vi "cb_mouseDblCk.vi"(4 "user param":refnum<vi>[](array[refnum]), 5 "이벤트 데이터":cluster{"sender":refnum<k24>, "e":refnum<k24>}, 6 "컨트롤 참조":refnum<k24>, 7 "이벤트 일반 데이터":cluster{"이벤트 소스":i32, "이벤트 타입":u32, "타임스탬프":u32}) -> ()   [LabVIEW 2019]
uses:
  dll/GMap.NET.WindowsForms.dll
  System.Windows.Forms
  gmap_fgv-cmd.ctl
  marker_info.ctl
  dll/GMap.NET.Core.dll
  System.Drawing
panel:
  out "type":i32(ring)=32 items=["none", "arrow", "blue", "blue_small", "blue_dot", "blue_pushpin", "brown_small", "gray_small", "green", "green_small", "green_dot", "green_pushpin", "green_big_go", "yellow", "yellow_small", "yellow_dot", "yellow_big_pause", "yellow_pushpin", "lightblue", "lightblue_dot", "lightblue_pushpin", "orange", "orange_small", "orange_dot", "pink", "pink_dot", "pink_pushpin", "purple", "purple_small", "purple_dot", "purple_pushpin", "red", "red_small", "red_dot", "red_pushpin", "red_big_stop", "black_small", "white_small"]
  out "Contains":bool
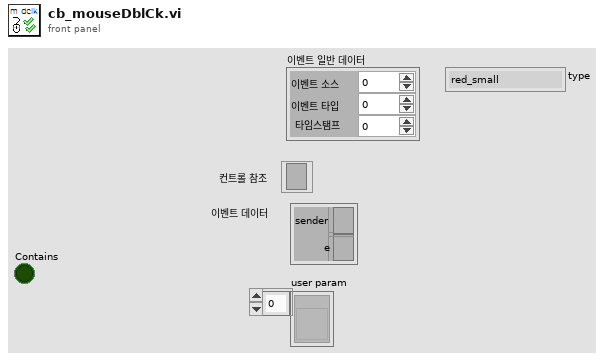
[diagram p1: front panel]
types:
  T1 = typedef "marker_info.ctl" = cluster{"arrLatLngActv":dbl[], "type":i32}
  T2 = typedef "gmap_fgv-cmd.ctl" = enum16{"marker type change", "save_image", "coll of points", "zoom n center markers", "add overlay reference", "read", "zoom", "set position by keyword", "set map provider", "map provider update", "create", "add marker", "clear marker", "close"}
  T3 = cluster{"MouseLat":refnum<vi>, "MouseLog":refnum<vi>, "MouseLat_DbClk":refnum<vi>, "MouseLog_DbClk":refnum<vi>, "PinDropLat_DblClk":refnum<vi>, "zoom":refnum<vi>}
  T4 = enum16{"none", "arrow", "blue", "blue_small", "blue_dot", "blue_pushpin", "brown_small", "gray_small", "green", "green_small", "green_dot", "green_pushpin", "green_big_go", "yellow", "yellow_small", "yellow_dot", "yellow_big_pause", "yellow_pushpin", "lightblue", "lightblue_dot", "lightblue_pushpin", "orange", "orange_small", "orange_dot", "pink", "pink_dot", "pink_pushpin", "purple", "purple_small", "purple_dot", "purple_pushpin", "red", "red_small", "red_dot", "red_pushpin", "red_big_stop", "black_small", "white_small"}
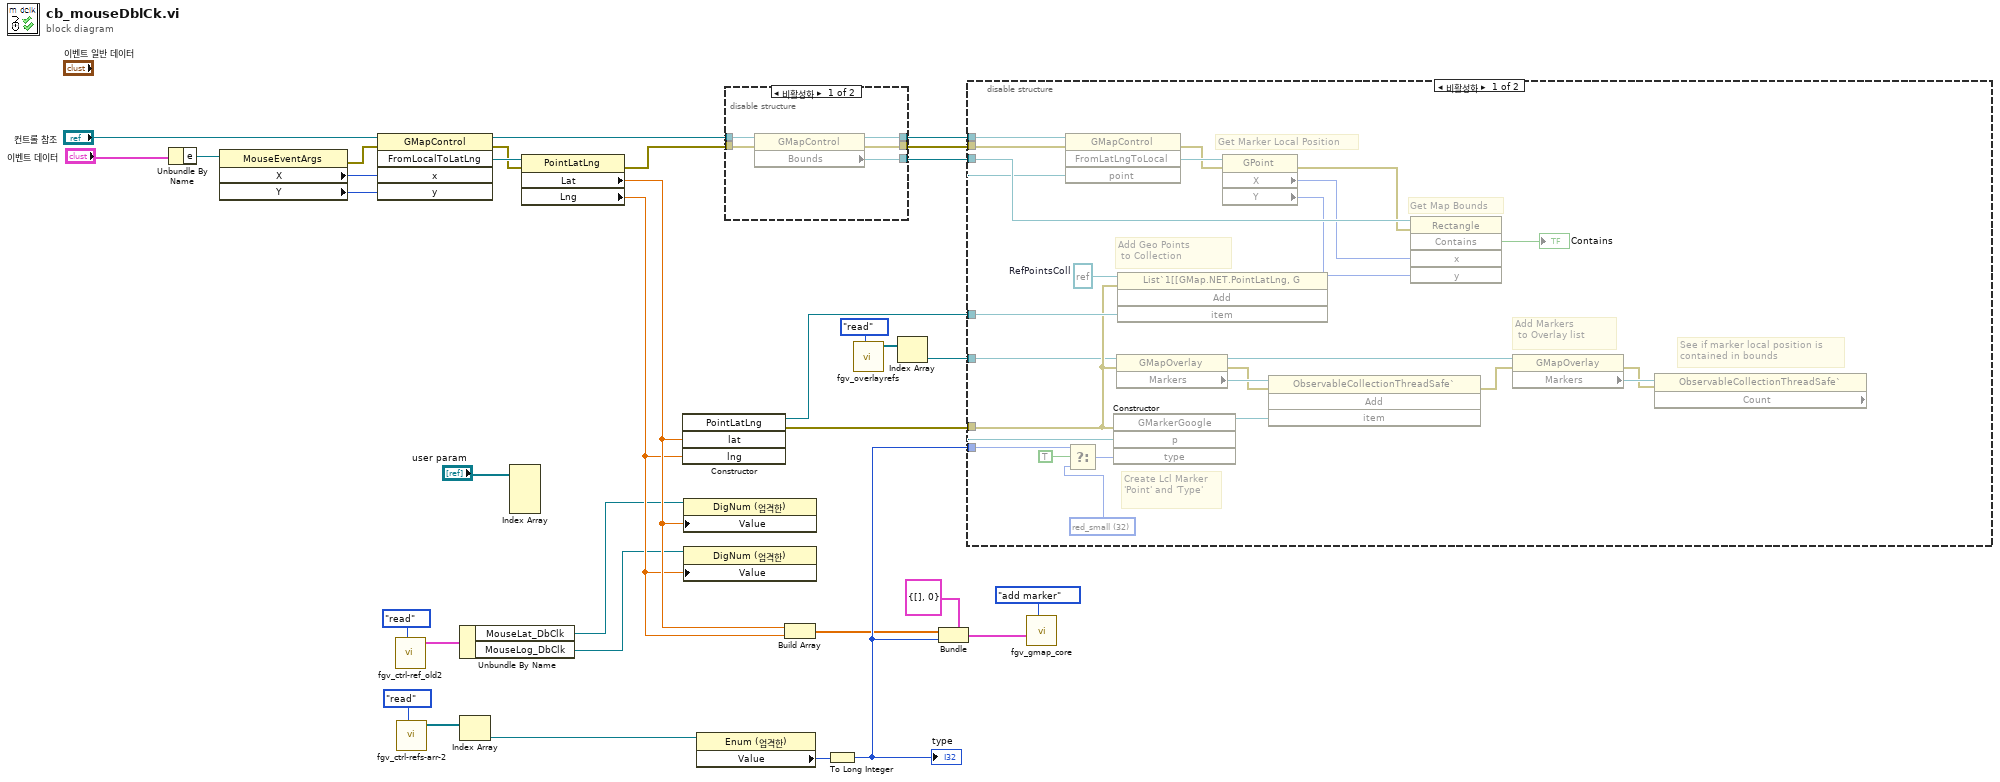
[diagram p0: block diagram]
diagram:
  n1 = Unbundle By Name("이벤트 데이터") -> ("e"=w24:refnum<k24>)
  n2 = property class="MouseEventArgs"(reference=w24) -> (error out=w20:errorcluster, "X"=w26:i32, "Y"=w25:i32)  [unwired: 1 in, 1 out]
  n3 = invoke class="GMapControl" method="FromLocalToLatLng"(reference="컨트롤 참조", error in=w20, "x"=w26, "y"=w25) -> (reference out=w17:refnum<k24>, error out=w19:errorcluster, "FromLocalToLatLng"=w23:refnum<k24>)  [unwired: 1 in, 2 out]
  n4 = call "fgv_ctrl-ref_old2.vi"("cmd"=enum16{"read", "write"}."read") -> ("ref out"=w1:T3)  [unwired: 10 in]
  n5 = call "fgv_ctrl-refs-arr-2.vi"("cmd"=enum16{"read", "write"}."read") -> ("ref out"=w4:refnum<vi>[])  [unwired: 10 in]
  n6 = Unbundle By Name(w1) -> ("MouseLat_DbClk"=w7:refnum<vi>, "MouseLog_DbClk"=w6:refnum<vi>)
  n7 = Index Array(array=w4) -> (element=w3:refnum<vi>)  [unwired: 1 in]
  n8 = Index Array(array="user param") -> ()  [unwired: 4 in, 4 out]
  n9 = property class="PointLatLng"(reference=w23, error in=w19) -> (error out=w18:errorcluster, "Lat"=w11:dbl, "Lng"=w10:dbl)  [unwired: 1 out]
  n10 = constructor class="PointLatLng"("lat"=w11, "lng"=w10) -> (reference out=w30:refnum<k24>, error out=w29:errorcluster)  [unwired: 3 in, 3 out]
  n11 = property class="DigNum (엄격한)"(reference=w7, "Value"=w11) -> ()  [unwired: 1 in, 2 out]
  n12 = property class="DigNum (엄격한)"(reference=w6, "Value"=w10) -> ()  [unwired: 1 in, 2 out]
  n13 = property class="Enum (엄격한)"(reference=w3) -> ("Value"=w15:T4)  [unwired: 1 in, 2 out]
  n14 = disable-structure shown="비활성화" {
    disable-tunnel: [w39 _] -> w33
    disable-tunnel: [w38 _] -> w32
    disable-tunnel: [w37 _] -> w31
    disable-tunnel: w18 -> [w36 _]
    disable-tunnel: w17 -> [w35 _]
    frame Disabled {
      n15 = property class="GMapControl"(reference=w35, error in=w36) -> (reference out=w38:refnum<k24>, error out=w37:errorcluster, "Bounds"=w39:refnum<k24>)
    }
    frame Enabled {
    }
  }
  n16 = Build Array(w11, w10) -> (w9:dbl[])
  n17 = To Long Integer(number=w15) -> (32bit integer=w13:i32)
  "type" <- w13
  n18 = call "fgv_overlayrefs.vi"("cmd"=enum16{"read", "write"}."read") -> ("overlayrefs out"=w28:refnum<k24>[])  [unwired: 10 in]
  n19 = Index Array(array=w28) -> (element=w27:refnum<k24>)  [unwired: 1 in]
  n20 = Bundle(cluster=T1 {"arrLatLngActv"=[], "type"=0} ("marker_info"), "arrLatLngActv"=w9, "type"=w13) -> (w12:T1)
  n21 = disable-structure shown="비활성화" {
    disable-tunnel: w33 -> [w59 _]
    disable-tunnel: w32 -> [w54 _]
    disable-tunnel: w31 -> [w53 _]
    disable-tunnel: w30 -> [w49 _]
    disable-tunnel: w29 -> [w45 _]
    disable-tunnel: w27 -> [w44 _]
    disable-tunnel: w13 -> [w42 _]
    frame Disabled {
      w43 = 32 items=["none", "arrow", "blue", "blue_small", "blue_dot", "blue_pushpin", "brown_small", "gray_small", "green", "green_small", "green_dot", "green_pushpin", "green_big_go", "yellow", "yellow_small", "yellow_dot", "yellow_big_pause", "yellow_pushpin", "lightblue", "lightblue_dot", "lightblue_pushpin", "orange", "orange_small", "orange_dot", "pink", "pink_dot", "pink_pushpin", "purple", "purple_small", "purple_dot", "purple_pushpin", "red", "red_small", "red_dot", "red_pushpin", "red_big_stop", "black_small", "white_small"] ("type")
      w63 = refnum<k24> refnum  # RefPointsColl
      # "See if marker local position is \ncontained in bounds"
      # "Get Marker Local Position"
      # "Get Map Bounds"
      # "Add Markers\n to Overlay list"
      # "Create Lcl Marker  'Point' and 'Type'"
      # "Add Geo Points\n to Collection"
      n22 = invoke class="GMapControl" method="FromLatLngToLocal"(reference=w54, error in=w53, "point"=w49) -> (error out=w52:errorcluster, "FromLatLngToLocal"=w57:refnum<k24>)  [unwired: 1 in, 2 out]
      n23 = Select(t=w42, s=TRUE, f=w43) -> (s? t:f=w40:i32)
      n24 = constructor class="GMarkerGoogle"(error in=w45, "p"=w49, "type"=w40) -> (reference out=w58:refnum<k24>)  [unwired: 2 in, 4 out]
      n25 = property class="GMapOverlay"(reference=w44, error in=w45) -> (reference out=w61:refnum<k24>, error out=w48:errorcluster, "Markers"=w60:refnum<k24>)
      n26 = invoke class="List`1[[GMap.NET.PointLatLng, G" method="Add"(reference=w63, error in=w45, "item"=w49) -> ()  [unwired: 1 in, 4 out]
      n27 = property class="GPoint"(reference=w57, error in=w52) -> (error out=w51:errorcluster, "X"=w56:i64, "Y"=w55:i64)  [unwired: 1 out]
      n28 = invoke class="ObservableCollectionThreadSafe`" method="Add"(reference=w60, error in=w48, "item"=w58) -> (error out=w47:errorcluster)  [unwired: 1 in, 3 out]
      n29 = invoke class="Rectangle" method="Contains"(reference=w59, error in=w51, "x"=w56, "y"=w55) -> ("Contains"=→"Contains":bool)  [unwired: 1 in, 4 out]
      n30 = property class="GMapOverlay"(reference=w61, error in=w47) -> (error out=w46:errorcluster, "Markers"=w62:refnum<k24>)  [unwired: 1 out]
      n31 = property class="ObservableCollectionThreadSafe`" props=["Count"](reference=w62, error in=w46) -> ()  [unwired: 3 out]
    }
    frame Enabled {
    }
  }
  n32 = call "fgv_gmap_core.vi"("cmd"=gmap_fgv-cmd."add marker", "marker_info"=w12) -> ()  [unwired: 6 in, 4 out]
